vi "Init HTTP TCP.vi"(8 "error in (no error)":errorcluster, 11 "LV Server in":refnum<class "LV Server.lvclass">) -> (0 "error out":errorcluster, 3 "LV Server out":refnum<class "LV Server.lvclass">)   [LabVIEW 2020, in "LV Server.lvclass"]
uses:
  LV Server.lvclass
  LV Server.lvclass/LV Server.ctl
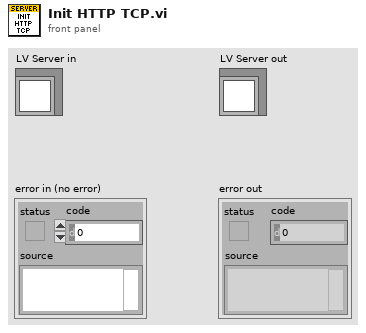
[diagram p1: front panel]
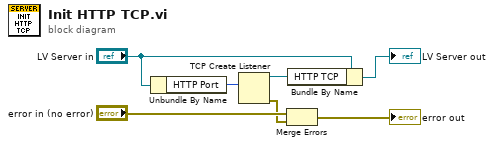
[diagram p0: block diagram]
diagram:
  n1 = Unbundle By Name("LV Server in") -> ("HTTP Port"=w5:u16)
  n2 = TCP Create Listener(10:w5) -> (0:w3:errorcluster, 3:w1:refnum<k5>)  [unwired: 4 in, 1 out]
  n3 = Merge Errors("error in (no error)", w3) -> (→"error out":errorcluster)
  n4 = Bundle By Name(cluster="LV Server in", "HTTP TCP"=w1) -> (→"LV Server out":refnum<class "LV Server.lvclass">)
